vi "CompareInitConfig(ExpertMode).vi"(10 "ExpertMode - existing":u32[](array[ring]) items=["FDX_EXPERT_MODE", "FDX_DISA_GHOST"], 11 "ExpertMode - new":T1 {"Expert1Mode" items=["FDX_EXPERT_MODE", "FDX_DISA_GHOST"]; "Expert2Mode" items=["FDX_EXPERT_MODE", "FDX_DISA_GHOST"]; "Expert3Mode" items=["FDX_EXPERT_MODE", "FDX_DISA_GHOST"]; "Expert4Mode" items=["FDX_EXPERT_MODE", "FDX_DISA_GHOST"]}) -> (2 "not equal":bool, 3 "ExpertMode - out":T1 {"Expert1Mode" items=["FDX_EXPERT_MODE", "FDX_DISA_GHOST"]; "Expert2Mode" items=["FDX_EXPERT_MODE", "FDX_DISA_GHOST"]; "Expert3Mode" items=["FDX_EXPERT_MODE", "FDX_DISA_GHOST"]; "Expert4Mode" items=["FDX_EXPERT_MODE", "FDX_DISA_GHOST"]})   [LabVIEW 2020, in "AIM664LV.lvlib"]
uses:
  AIM664LV.lvlib
  _controls/initialize_ExpertMode.ctl
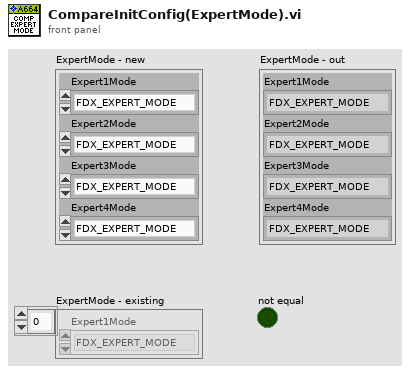
[diagram p1: front panel]
types:
  T1 = typedef "AIM664LV.lvlib/initialize_ExpertMode.ctl" = cluster{"Expert1Mode":u32, "Expert2Mode":u32, "Expert3Mode":u32, "Expert4Mode":u32}
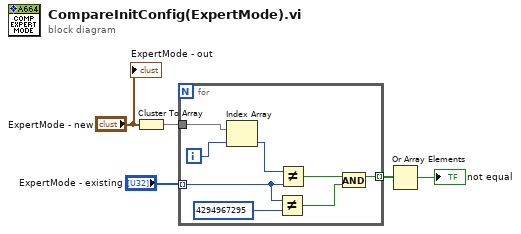
[diagram p0: block diagram]
diagram:
  n1 = Cluster To Array(cluster="ExpertMode - new") -> (array=w3:u32[])
  n2 = for {
    tunnel: "ExpertMode - existing" -> [w9] mode=indexing
    tunnel: w3 -> [w13]
    tunnel: [w7] -> w1 mode=indexing
    i -> [w12]
    n3 = Index Array(array=w13, index=w12) -> (element=w11:u32)
    n4 = Not Equal?(x=w9, y=u32 4294967295) -> (x != y?=w6:bool)
    n5 = Not Equal?(x=w11, y=w9) -> (x != y?=w10:bool)
    n6 = And(x=w10, y=w6) -> (x .and. y?=w7:bool)
  }
  n7 = Or Array Elements(Boolean array=w1) -> (logical OR=→"not equal":bool)
  "ExpertMode - out" <- "ExpertMode - new"
